vi "Read Macro Config.vi"(8 "error in (no error)":errorcluster, 11 "refnum":T4) -> (0 "error out":errorcluster, 1 "Macro (Config Only)":T1, 2 "Schema Version":string, 3 "refnum out":T4)   [LabVIEW 2023]
doc: "Loads the macro defined by <B>Macro Name</B> from the config file defined by <B>refnum</B>."
uses:
  <vilib>/Utility/config.llb/Config Data RefNum.ctl
  CTLs/Macro Cluster V3.ctl
  CTLs/Step V3.ctl
  CTLs/Step Type V3.ctl
  <vilib>/Utility/config.llb/Read Key (String).vi
  <vilib>/Utility/config.llb/Read Key (U32).vi
  <vilib>/Utility/config.llb/Read Key (I32).vi
  <vilib>/Utility/error.llb/Error Cluster From Error Code.vi
  <vilib>/ErrorRing/Error Ring.xnode
  <vilib>/Utility/config.llb/NI_LVConfig.lvlib
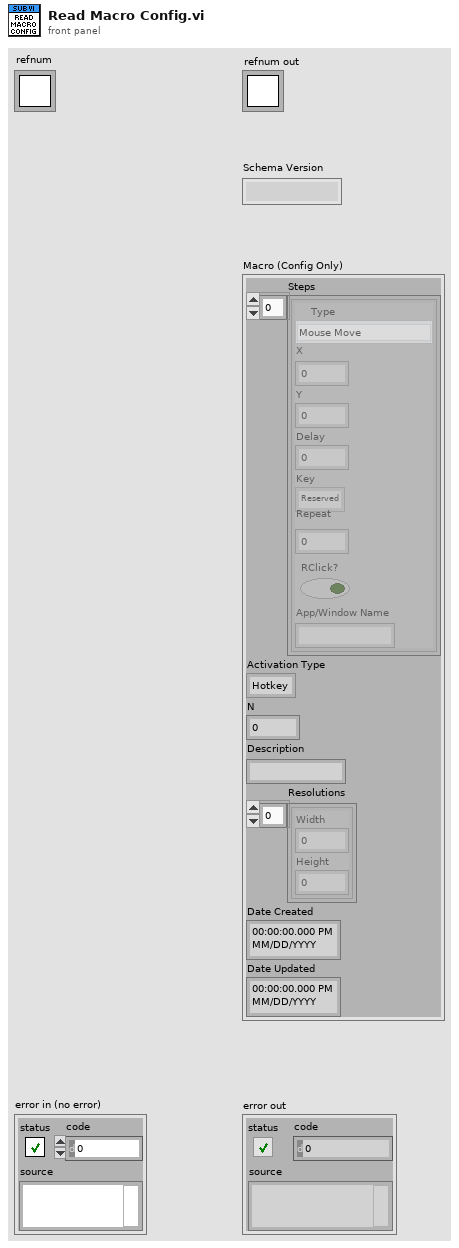
[diagram p1: front panel]
types:
  T1 = typedef "Macro Cluster V3.ctl" = cluster{"Steps":T2[], "Activation Type":enum32{"Hotkey", "Automatic"}, "N":i32, "Description":string, "Resolutions":cluster{"Width":i16, "Height":i16}[], "Date Created":timestamp, "Date Updated":timestamp}
  T2 = typedef "Step V3.ctl" = cluster{"Type":T3, "X":i32, "Y":i32, "Delay":i32, "Key":u8, "Repeat":i32, "RClick?":bool, "App/Window Name":string}
  T3 = typedef "Step Type V3.ctl" = enum16{"Mouse Move", "Mouse Click", "Key Press", "Wait", "Mouse Down", "Mouse Up", "Key Down", "Key Up", "Run Application", "Quit Application", "Maximize Window", "Minimize Window", "Bring Window to Front", "Send Window to Back"}
  T4 = typedef "NI_LVConfig.lvlib/Config Data RefNum.ctl" = refnum<k1>
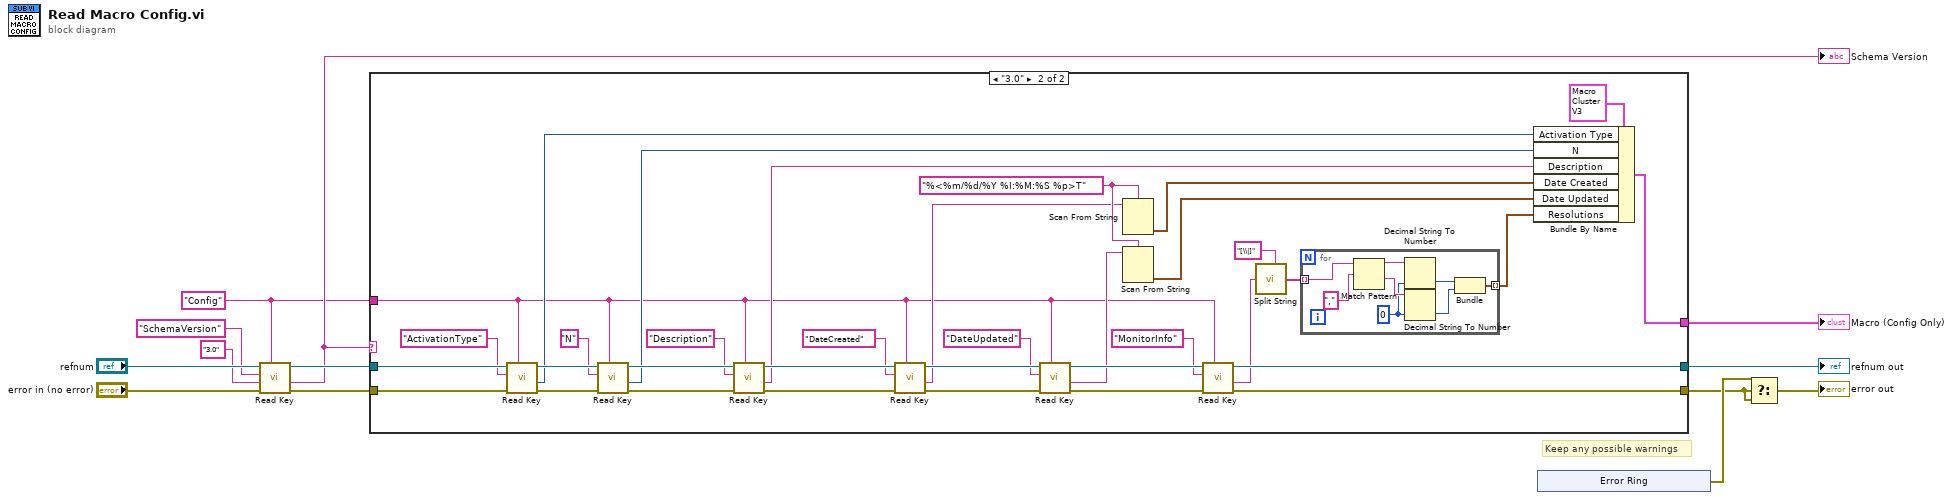
[diagram p0: block diagram]
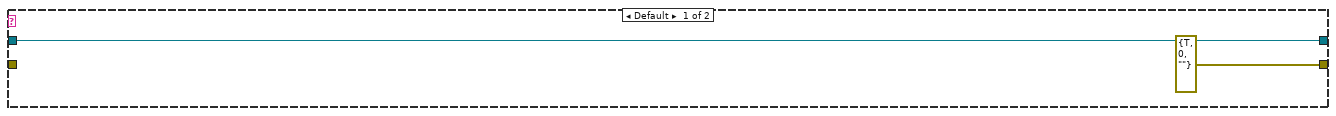
[diagram p2: hidden frame]
diagram:
  w5 = "Config" ("section")
  # "Keep any possible warnings"
  n1 = call-poly <vilib>:"Read Key.vi"("section"=w5, "error in (no error)"="error in (no error)", "default value"="3.0", "key"="SchemaVersion", "refnum"="refnum") -> ("error out"=w9:errorcluster, "value"=w6:string, "refnum out"=w10:T4)  [unwired: 3 in, 1 out]
  "Schema Version" <- w6
  n2 = case shown="\"3.0\"" w6 {
    tunnel: w10 -> [w15 w50]
    tunnel: [w15 w22] -> w3
    tunnel: w9 -> [_ w43]
    tunnel: w5 -> [_ w16]
    tunnel: [errorcluster {"status"=TRUE, "code"=0, "source"=""} ("error out") w21] -> w2
    tunnel: [_ w42] -> w1
    frame Default {
    }
    frame "3.0" {
      w31 = "%<%m/%d/%Y %I:%M:%S %p>T" ("format string")
      n3 = call-poly <vilib>:"Read Key.vi"("section"=w16, "error in (no error)"=w43, "key"="ActivationType", "refnum"=w50) -> ("error out"=w39:errorcluster, "value"=w34:u32, "refnum out"=w49:T4)  [unwired: 4 in, 1 out]
      n4 = call-poly <vilib>:"Read Key.vi"("section"=w16, "error in (no error)"=w39, "key"="N", "refnum"=w49) -> ("error out"=w37:errorcluster, "value"=w33:i32, "refnum out"=w48:T4)  [unwired: 4 in, 1 out]
      n5 = call-poly <vilib>:"Read Key.vi"("section"=w16, "error in (no error)"=w37, "key"="Description", "refnum"=w48) -> ("error out"=w35:errorcluster, "value"=w32:string, "refnum out"=w47:T4)  [unwired: 4 in, 1 out]
      n6 = call-poly <vilib>:"Read Key.vi"("section"=w16, "error in (no error)"=w35, "key"="DateCreated", "refnum"=w47) -> ("error out"=w27:errorcluster, "value"=w25:string, "refnum out"=w46:T4)  [unwired: 4 in, 1 out]
      n7 = call-poly <vilib>:"Read Key.vi"("section"=w16, "error in (no error)"=w27, "key"="DateUpdated", "refnum"=w46) -> ("error out"=w23:errorcluster, "value"=w24:string, "refnum out"=w45:T4)  [unwired: 4 in, 1 out]
      n8 = Scan From String(format string=w31, input string=w25) -> (output 1=w30:timestamp)  [unwired: 3 in, 3 out]
      n9 = Scan From String(format string=w31, input string=w24) -> (output 1=w29:timestamp)  [unwired: 3 in, 3 out]
      n10 = call-poly <vilib>:"Read Key.vi"("section"=w16, "error in (no error)"=w23, "key"="MonitorInfo", "refnum"=w45) -> ("error out"=w21:errorcluster, "value"=w18:string, "refnum out"=w22:T4)  [unwired: 4 in, 1 out]
      n11 = call <vilib>:"Split String.vi"("Split Pattern"="[\\|]", "Input String"=w18) -> ("Split String"=w20:string[])  [unwired: 5 in]
      n12 = for {
        tunnel: w20 -> [w58] mode=indexing
        tunnel: [w52] -> w17 mode=indexing
        w51 = i16 0 ("default (0 I32)")
        n13 = Match Pattern(string=w58, regular expression=",") -> (before substring=w56:string, after substring=w55:string)  [unwired: 1 in, 2 out]
        n14 = Decimal String To Number(string=w56, default (0L)=w51) -> (number=w54:i16)  [unwired: 1 in, 1 out]
        n15 = Decimal String To Number(string=w55, default (0L)=w51) -> (number=w53:i16)  [unwired: 1 in, 1 out]
        n16 = Bundle(w54, w53) -> (w52:cluster{i16, i16})  [unwired: 1 in]
      }
      n17 = Bundle By Name(cluster=T1 {"Steps"=[], "Activation Type"=enum."Hotkey", "N"=0, "Description"="", "Resolutions"=[], "Date Created"=timestamp(0 s since 1904-01-01), "Date Updated"=timestamp(0 s since 1904-01-01)} ("Macro Cluster"), "Activation Type"=w34, "N"=w33, "Description"=w32, "Date Created"=w30, "Date Updated"=w29, "Resolutions"=w17) -> (w42:T1)
    }
  }
  "refnum out" <- w3
  "Macro (Config Only)" <- w1
  n18 = xnode "Error Ring"() -> ("error out"=w12:errorcluster)
  n19 = Select(t=w12, s=w2, f=w2) -> (s? t:f=→"error out":errorcluster)
